vi "Beam_flicker_for_perimetry.vi"(8 "shiftY":dbl, 9 "shiftX":dbl) -> (0 "Rate":dbl=12800.0, 2 "Scanners trajectories":dbl[][](graph), 3 "XY Graph":cluster{dbl[], dbl[]}(graph))   [LabVIEW 2021]
uses:
  <vilib>/Analysis/1siggen.llb/Ramp Pattern by Samples.vi
  <vilib>/Analysis/NI_AALBase.lvlib
panel:
  out "output array":dbl[][](array[numeric])
  in  "Number of cycles":i32=20
  # "Ta wersja Flicker beam zakłada,  ze skanery są cały czas w tle (x = 0V, Y = -4V), wyprowadza je z tła i kończy w tle."
  # "Przy 12800 S/s i 128 sampli na bodziec, czas trwania 1 cyklu 10 ms"
  # "przerwa w tle ustawiona na 600 ms"
  # "Dodatkowo najazdy trwają 2 razy po 1,5 ms"
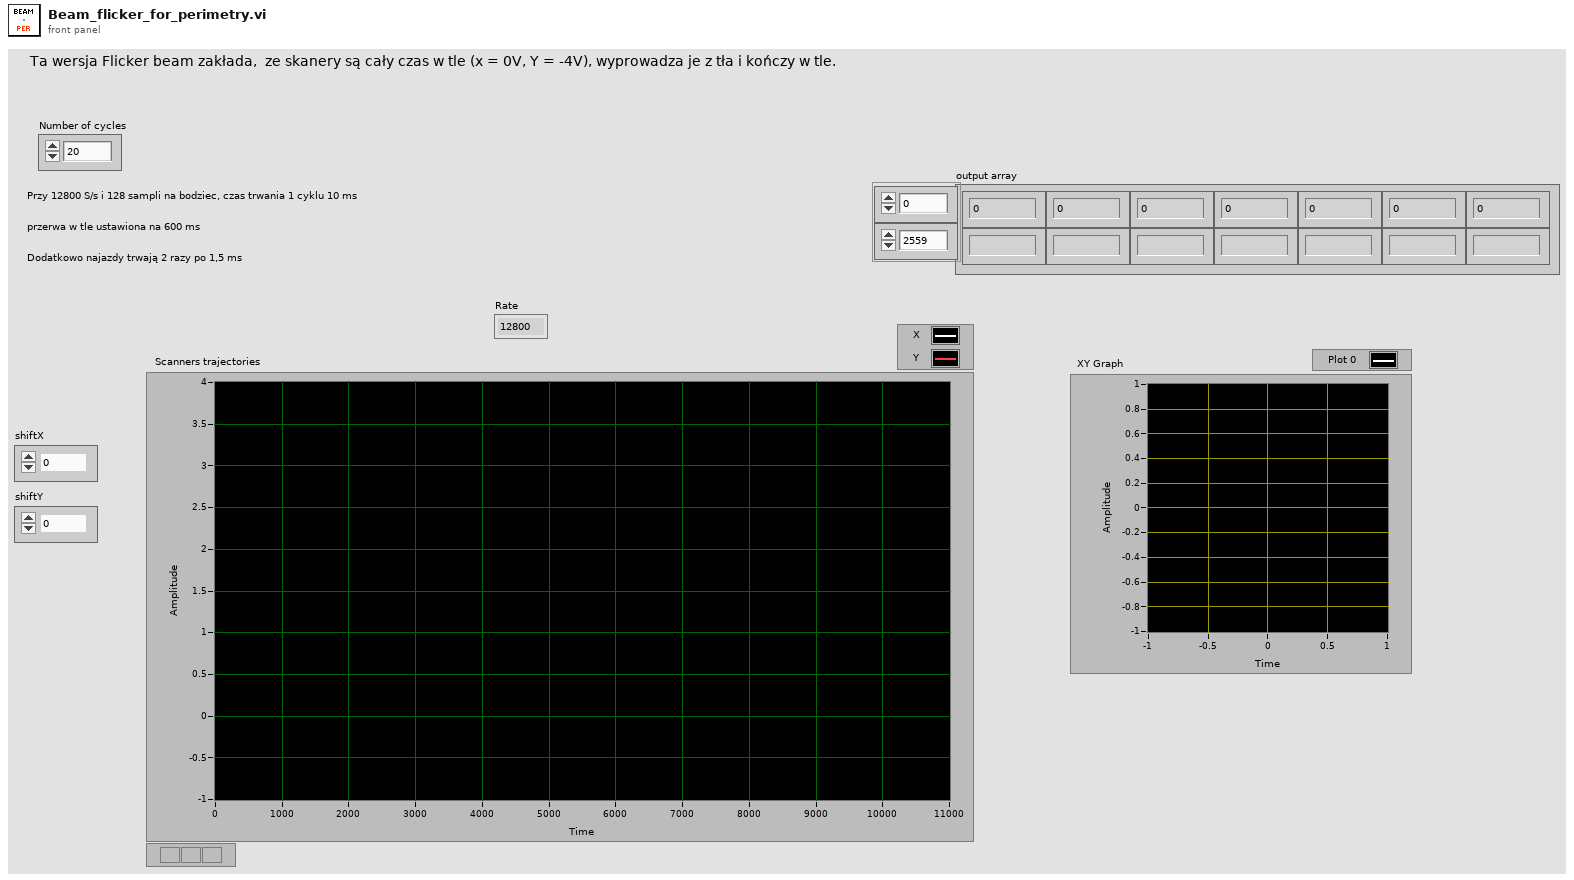
[diagram p1: front panel]
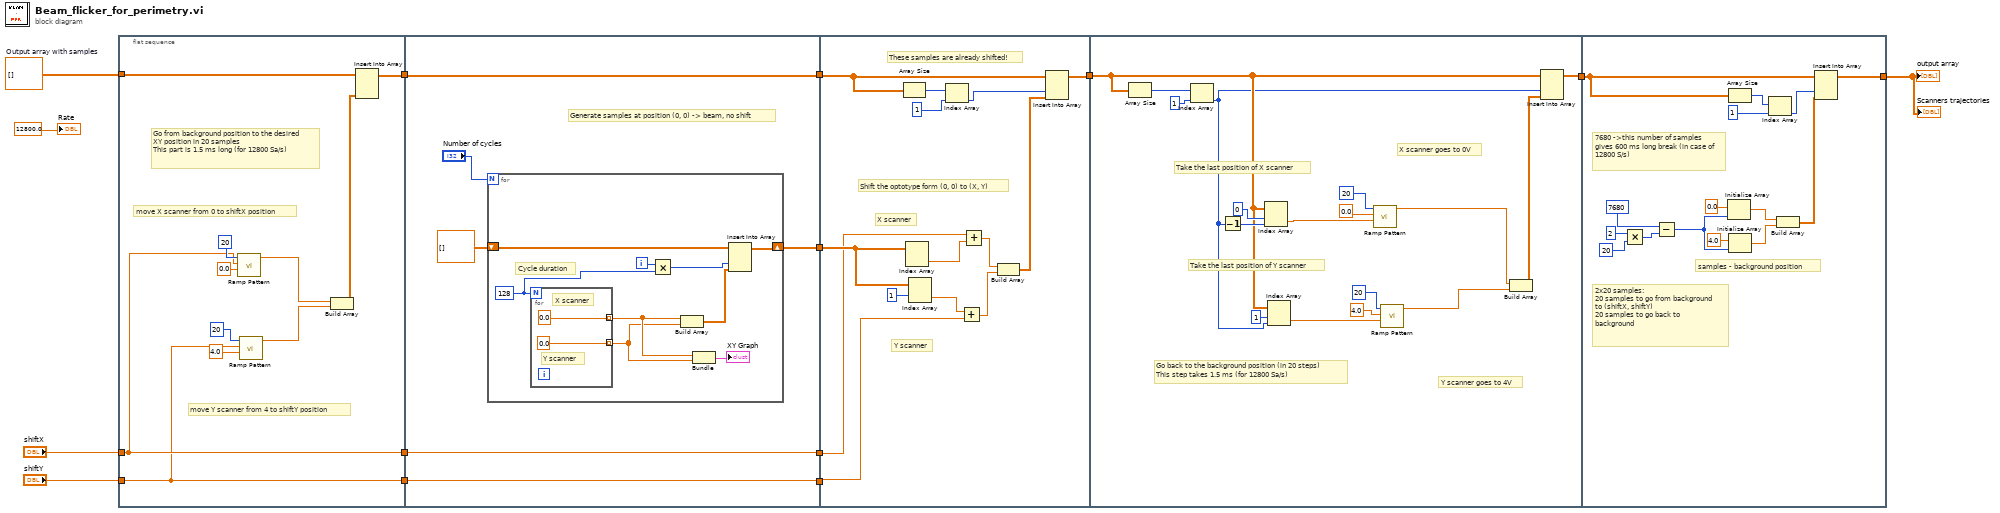
[diagram p0: block diagram]
diagram:
  w10 = dbl[][] []  # Output array with samples
  n1 = flat-sequence {
    tunnel: w10 -> [w22]
    tunnel: [w19] -> w9
    tunnel: [w16] -> w7
    tunnel: "shiftX" -> [w16]
    tunnel: [w15] -> w5
    tunnel: "shiftY" -> [w15]
    tunnel: [w26] -> w12
    tunnel: w9 -> [w30]
    tunnel: [w30] -> w8
    tunnel: w7 -> [w29]
    tunnel: w5 -> [w28]
    tunnel: [w29] -> w3
    tunnel: [w28] -> w2
    tunnel: w12 -> [w51]
    tunnel: [w50] -> w11
    tunnel: w8 -> [w46]
    tunnel: w3 -> [w43]
    tunnel: w2 -> [w44]
    tunnel: w11 -> [w60]
    tunnel: [w68] -> w14
    tunnel: w14 -> [w78]
    tunnel: [w74] -> w1
    frame #0 {
      # "move Y scanner from 4 to shiftY position"
      # "move X scanner from 0 to shiftX position"
      # "Go from background position to the desired XY position in 20 samples\nThis part is 1.5 ms long (for 12800 Sa/s)"
      n2 = call-poly <vilib>:"Ramp Pattern.vi"("start"=0.0 ("element"), "end"=w16, "samples"=20) -> ("Ramp Pattern"=w23:dbl[])  [unwired: 7 in, 1 out]
      n3 = call-poly <vilib>:"Ramp Pattern.vi"("start"=4.0 ("end"), "end"=w15, "samples"=20) -> ("Ramp Pattern"=w25:dbl[])  [unwired: 7 in, 1 out]
      n4 = Build Array(w23, w25) -> (w24:dbl[][])
      n5 = Insert Into Array(array=w22, new element=w24) -> (w19:dbl[][])  [unwired: 2 in]
    }
    frame #1 {
      # "Generate samples at position (0, 0) -> beam, no shift"
      n6 = for {
        N: "Number of cycles" -> [_]
        shift-right: [w40] -> w26
        shift-left: dbl[][] [] -> [w39]
        i -> [w38]
        w37 = 128
        # "Cycle duration"
        n7 = for {
          N: w37 -> [_]
          tunnel: [0.0] -> w34 mode=indexing
          tunnel: [0.0] -> w33 mode=indexing
          # "X scanner"
          # "Y scanner"
        }
        n8 = Multiply(x=w38, y=w37) -> (x*y=w36:i32)
        n9 = Build Array(w34, w33) -> (w32:dbl[][])
        n10 = Bundle(w34, w33) -> (→"XY Graph":cluster{dbl[], dbl[]})  [unwired: 1 in]
        n11 = Insert Into Array(array=w39, index (col)=w36, new element=w32) -> (w40:dbl[][])  [unwired: 1 in]
      }
    }
    frame #2 {
      # "Y scanner"
      # "X scanner"
      # "These samples are already shifted!"
      # "Shift the optotype form (0, 0) to (X, Y)"
      n12 = Array Size(array=w46) -> (size(s)=w48:i32[])
      n13 = Index Array(array=w51) -> (element=w53:dbl[])  [unwired: 2 in]
      n14 = Index Array(array=w51, index (row)=1) -> (element=w54:dbl[])  [unwired: 1 in]
      n15 = Index Array(array=w48, index=1) -> (element=w45:i32)
      n16 = Add(x=w54, y=w44) -> (x+y=w56:dbl[])
      n17 = Add(x=w43, y=w53) -> (x+y=w55:dbl[])
      n18 = Build Array(w55, w56) -> (w49:dbl[][])
      n19 = Insert Into Array(array=w46, index (col)=w45, new element=w49) -> (w50:dbl[][])  [unwired: 1 in]
    }
    frame #3 {
      # "X scanner goes to 0V"
      # "Y scanner goes to 4V"
      # "Go back to the background position (in 20 steps)\nThis step takes 1.5 ms (for 12800 Sa/s)"
      # "Take the last position of Y scanner"
      # "Take the last position of X scanner"
      n20 = Array Size(array=w60) -> (size(s)=w71:i32[])
      n21 = Index Array(array=w71, index=1) -> (element=w58:i32)
      n22 = Decrement(x=w58) -> (x-1=w64:i32)
      n23 = Index Array(array=w60, index (row)=0, index (col)=w64) -> (element=w63:dbl)
      n24 = Index Array(array=w60, index (row)=1, index (col)=w58) -> (element=w57:dbl)
      n25 = call-poly <vilib>:"Ramp Pattern.vi"("start"=w63, "end"=0.0 ("element"), "samples"=20) -> ("Ramp Pattern"=w61:dbl[])  [unwired: 7 in, 1 out]
      n26 = call-poly <vilib>:"Ramp Pattern.vi"("start"=w57, "end"=4.0, "samples"=20 ("dimension size")) -> ("Ramp Pattern"=w72:dbl[])  [unwired: 7 in, 1 out]
      n27 = Build Array(w61, w72) -> (w69:dbl[][])
      n28 = Insert Into Array(array=w60, index (col)=w58, new element=w69) -> (w68:dbl[][])  [unwired: 1 in]
    }
    frame #4 {
      # "2x20 samples:\n20 samples to go from background to (shiftX, shiftY)\n20 samples to go back to background"
      # "7680 ->this number of samples gives 600 ms long break (in case of 12800 S/s)"
      # "samples - background position"
      n29 = Multiply(x=2, y=20) -> (x*y=w82:i32)
      n30 = Subtract(x=7680 ("Numeric Control"), y=w82) -> (x-y=w81:i32)
      n31 = Initialize Array(0.0 ("element"), w81) -> (w86:dbl[])
      n32 = Array Size(array=w78) -> (size(s)=w80:i32[])
      n33 = Initialize Array(4.0 ("element"), w81) -> (w85:dbl[])
      n34 = Index Array(array=w80, index=1) -> (element=w77:i32)
      n35 = Build Array(w86, w85) -> (w76:dbl[][])
      n36 = Insert Into Array(array=w78, index (col)=w77, new element=w76) -> (w74:dbl[][])  [unwired: 1 in]
    }
  }
  "Scanners trajectories" <- w1
  "Rate" <- 12800.0 ("Rate")
  "output array" <- w1
